vi "create_full_endpoint.vi"(8 "error in (no error)":errorcluster, 11 "llm_azureopenai_chatmodels in":refnum<class "llm_azureopenai_chatmodels.lvclass">) -> (0 "error out":errorcluster, 2 "endpoint":string, 3 "llm_azureopenai_chatmodels out":refnum<class "llm_azureopenai_chatmodels.lvclass">)   [LabVIEW 2020, in "llm_azureopenai_chatmodels.lvclass"]
uses:
  llm_azureopenai_chatmodels.lvclass
  D:/Personal/LabVIEW LLMs/src/models/llm_openai_chatmodels/llm_openai_chatmodels.lvclass
  llm_azureopenai_chatmodels.lvclass/llm_azureopenai_chatmodels.ctl
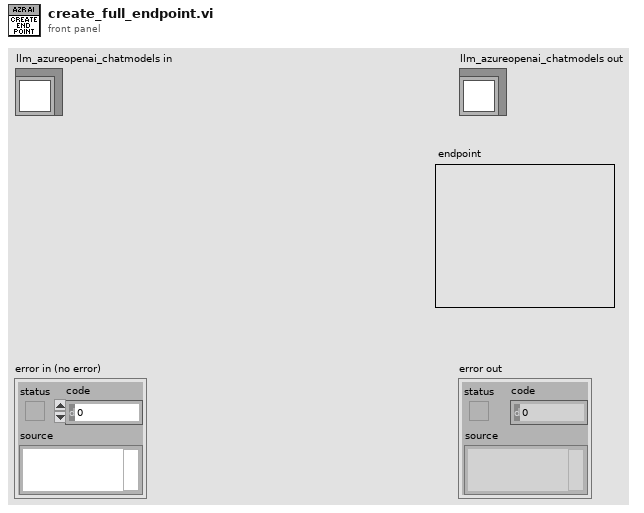
[diagram p1: front panel]
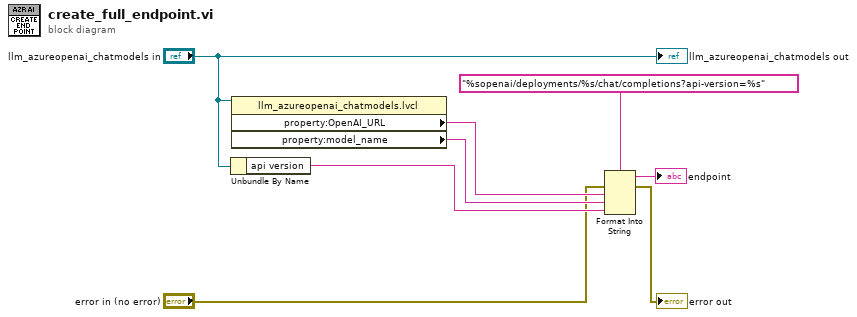
[diagram p0: block diagram]
diagram:
  n1 = Unbundle By Name("llm_azureopenai_chatmodels in") -> ("api version"=w7:string)
  n2 = property class="llm_azureopenai_chatmodels.lvcl"(reference="llm_azureopenai_chatmodels in") -> ("property:OpenAI_URL"=w5:string, "property:model_name"=w4:string)  [unwired: 1 in, 2 out]
  n3 = Format Into String(format string="%sopenai/deployments/%s/chat/completions?api-version=%s", error in="error in (no error)", w5, w4, w7) -> (resulting string=→"endpoint":string, error out=→"error out":errorcluster)  [unwired: 1 in]
  "llm_azureopenai_chatmodels out" <- "llm_azureopenai_chatmodels in"
